vi "Initialize Root.vi"(6 "RootQueueName":string, 8 "error in (no error)":errorcluster caption="错误输入（无错误）", 9 "CurrentVi*":refnum<vi>, 10 "RootPanel*":refnum<vi>, 11 "PCM MenuVIPanelSplit 输入":refnum<class "PCM MenuVIPanelSplit.lvclass"> caption="DNL_LabVIEW Object in") -> (0 "error out":errorcluster caption="错误输出", 2 "SelfNode*":refnum<data-value>)   [LabVIEW 2016, in "PCM MenuVIPanelSplit.lvclass"]
uses:
  PCM MenuVIPanelSplit.lvclass
  PanelSplitToolkit/PanelRootNode/PanelRootNode.lvclass
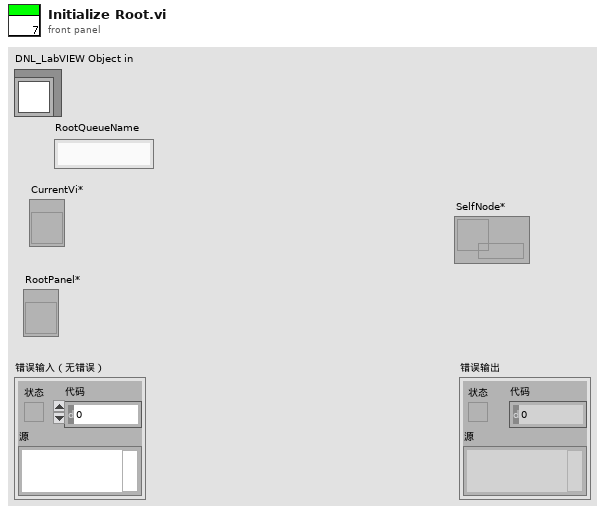
[diagram p1: front panel]
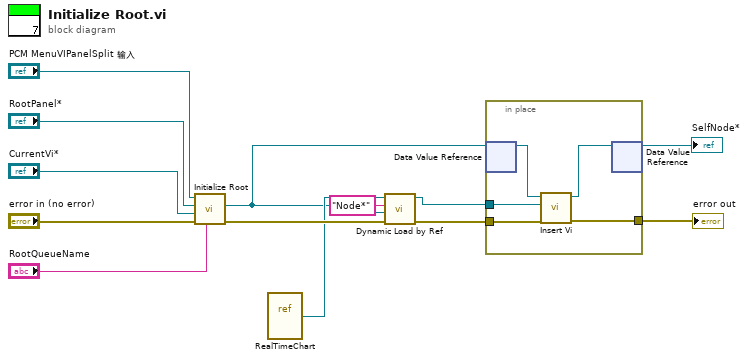
[diagram p0: block diagram]
diagram:
  n1 = call-parent "Initialize Root.vi"("RootQueueName"="RootQueueName", "error in (no error)"="error in (no error)", "CurrentVi*"="CurrentVi*", "RootPanel*"="RootPanel*", "PanelRootNode 输入"="PCM MenuVIPanelSplit 输入") -> ("error out"=w7:errorcluster, "SelfNode*"=w2:refnum<data-value>)  [unwired: 5 in]
  n2 = vi-ref "RealTimeChart.vi"() -> (w4:refnum<vi>)
  n3 = call "Dynamic Load by Ref.vi"("error in"=w7, "CtrlValue"=w2, "CtrlName"="Node*", "Static vi reference in"=w4) -> ("错误输出"=w6:errorcluster, "Dynamic vi reference out"=w5:refnum<vi>)  [unwired: 6 in]
  n4 = in-place {
    in-place-border: w6 -> [w15]
    in-place-border: [w18] -> w9
    in-place-border: w5 -> [w14]
    n5 = in-place-dvr #1(w2) -> (w17:refnum<class "PanelRootNode.lvclass">)  [unwired: 1 out]
    n6 = call-dynamic "Insert Vi.vi"("error in (no error)"=w15, "VI*"=w14, "PanelDataNode 输入"=w17) -> ("error out"=w18:errorcluster, "PanelDataNode 输出"=w16:refnum<class "PanelRootNode.lvclass">)  [unwired: 7 in]
    n7 = in-place-dvr #1(w16) -> (→"SelfNode*":refnum<data-value>)  [unwired: 1 out]
  }
  "error out" <- w9
